vi "TestBodyIcon.vi"() -> ()   [LabVIEW 2020]
uses:
  resource/Framework/Providers/Open_GDS/ClassProviders/Common/LvIcon_class/GDSLvIcon_Type.ctl
panel:
  out "24-bit pixmap":u32[][](array[numeric]) format="%x"
  out "new picture 8":picture
  out "new picture 7":picture
  in  "ClassBodyIcon":string
  in  "Type":T1
  in  "Color Box 2":u32(colorbox)
  in  "_Thickness":u8=1 caption="Thickness (pixels)" min=1 max=3 step=1
  in  "Width(30)":u32=30
  in  "Height":u32=22
  out "new picture 6":picture
  out "new picture 5":picture
  in  "Color Box":u32(colorbox)
  out "number of rows":i32
  out "number of columns":i32
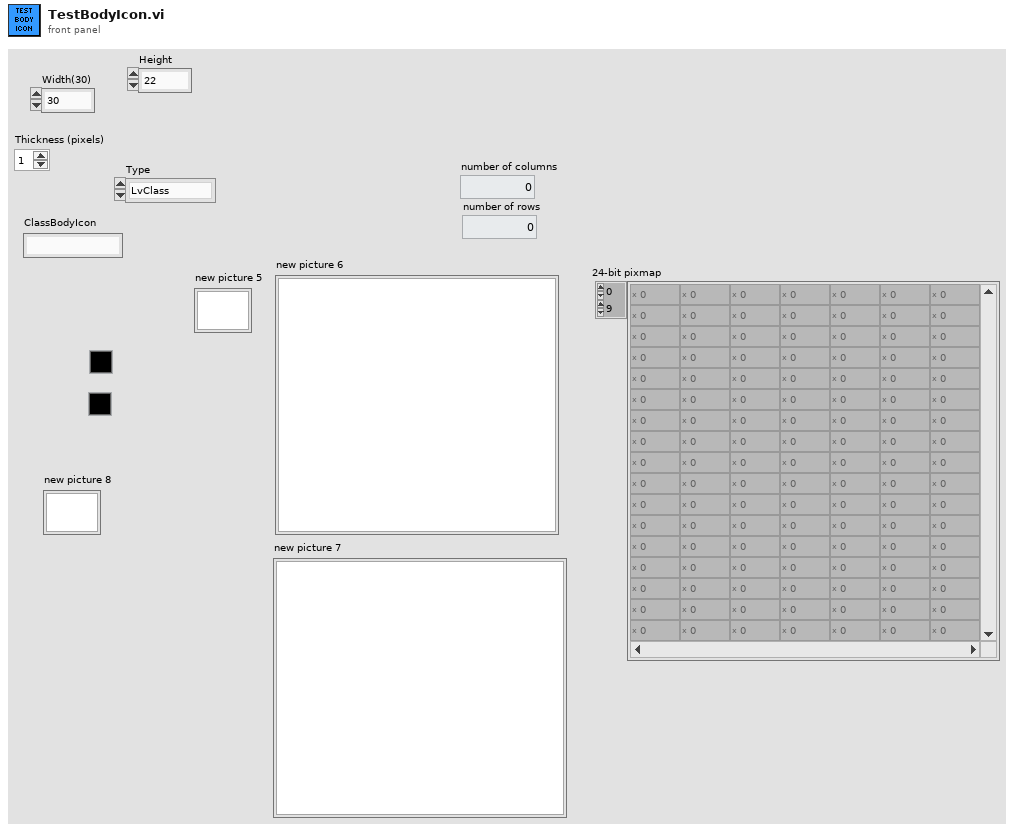
[diagram p1: front panel]
types:
  T1 = typedef "GDSLvIcon_Type.ctl" = enum16{"LvClass", "Library", "X-Control", "LvInterface"}
  T2 = typedef "imagedata.ctl" = cluster{"image type":i32, "image depth":i32, "image":u8[], "mask":u8[], "colors":u32[], "Rectangle":cluster{"left":i16, "top":i16, "right":i16, "bottom":i16}}
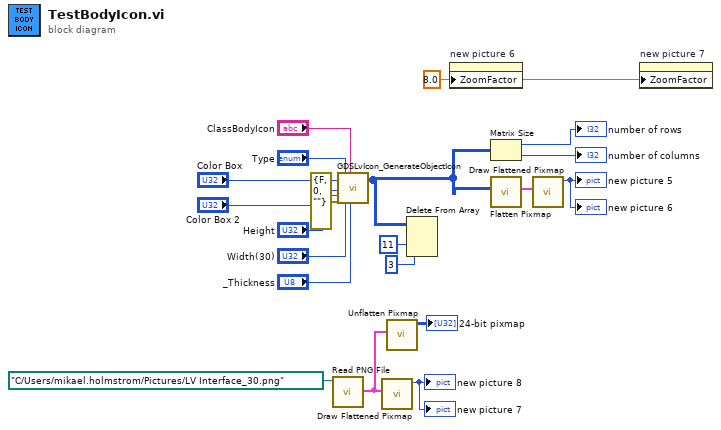
[diagram p0: block diagram]
diagram:
  w4 = sgl 8.0 ("Zoom Factor")
  n1 = call <vilib>:"Read PNG File.vi"("path to PNG file"=path "C:/Users/mikael.holmstrom/Pictures/LV Interface_30.png") -> ("image data"=w6:T2)  [unwired: 8 in, 2 out]
  n2 = call "GDSLvIcon_GenerateObjectIcon.vi"("HeaderColor"="Color Box", "BackgroundColor"="Color Box 2", "Height"="Height", "error in (no error)"=errorcluster {"status"=FALSE, "code"=0, "source"=""}, "Type"="Type", "Width(30)"="Width(30)", "ClassBodyIcon"="ClassBodyIcon", "_Thickness"="_Thickness") -> ("BodyIconOut"=w1:u8[][])  [unwired: 10 in, 1 out]
  n3 = call <vilib>:"Draw Flattened Pixmap.vi"("image data"=w6) -> ("new picture"=→"new picture 8" →"new picture 7":picture)  [unwired: 8 in]
  n4 = call <vilib>:"Unflatten Pixmap.vi"("image data"=w6) -> ("24-bit pixmap"=→"24-bit pixmap":u32[][])  [unwired: 4 in, 6 out]
  n5 = Delete From Array(array=w1, length=3, index (row)=11) -> ()  [unwired: 1 in, 2 out]
  n6 = property on="new picture 6" class="Pict"("ZoomFactor"=w4) -> ()  [unwired: 2 in, 2 out]
  n7 = Matrix Size(0:w1) -> (1:→"number of rows":i32, 2:→"number of columns":i32)
  n8 = call <vilib>:"Flatten Pixmap.vi"("8-bit pixmap"=w1) -> ("image data"=w18:T2)  [unwired: 10 in]
  n9 = call <vilib>:"Draw Flattened Pixmap.vi"("image data"=w18) -> ("new picture"=→"new picture 5" →"new picture 6":picture)  [unwired: 8 in]
  n10 = property on="new picture 7" class="Pict"("ZoomFactor"=w4) -> ()  [unwired: 2 in, 2 out]
